vi "Build Part Number from digit array.vi"(11 "Digit Array":T1[](array[typedef])) -> (3 "Part Number Out":i32)   [LabVIEW 2023]
uses:
  Cluster Digit.ctl
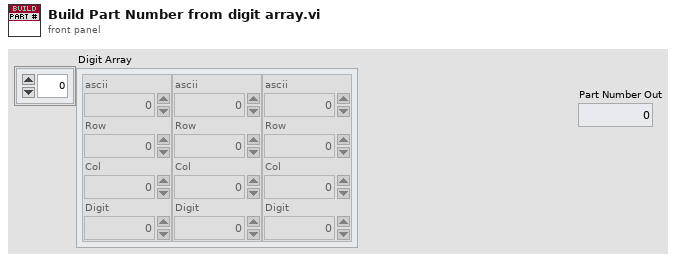
[diagram p1: front panel]
types:
  T1 = typedef "Cluster Digit.ctl" = cluster{"ascii":u8, "Row":i32, "Col":i32, "Digit":i32}
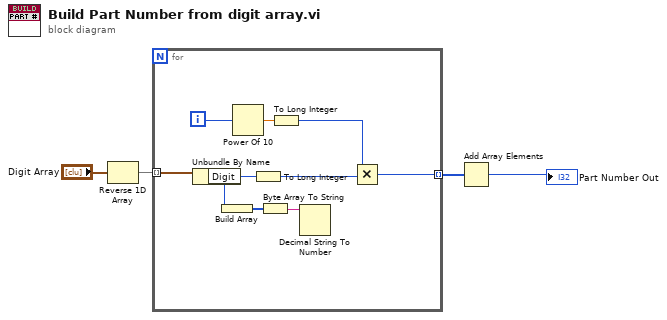
[diagram p0: block diagram]
diagram:
  n1 = Reverse 1D Array(array="Digit Array") -> (reversed array=w3:T1[])
  n2 = for {
    tunnel: w3 -> [w13] mode=indexing
    tunnel: [w10] -> w2 mode=indexing
    i -> [w12]
    n3 = Unbundle By Name(w13) -> ("Digit"=w7:i32)
    n4 = Build Array(w7) -> (w6:i32[])
    n5 = Power Of 10(x=w12) -> (10^x=w11:dbl)
    n6 = To Long Integer(number=w7) -> (32bit integer=w8:i32)
    n7 = Byte Array To String(unsigned byte array=w6) -> (string=w5:string)
    n8 = To Long Integer(number=w11) -> (32bit integer=w9:i32)
    n9 = Decimal String To Number(string=w5) -> ()  [unwired: 2 in, 2 out]
    n10 = Multiply(x=w9, y=w8) -> (x*y=w10:i32)
  }
  n11 = Add Array Elements(numeric array=w2) -> (sum=→"Part Number Out":i32)
